vi "Process Intiation Response.vi"(5 "password":string, 7 "user name":string, 8 "error in (no error)":errorcluster, 9 "publicKeyB":u8[](array[numeric]), 10 "salt":u8[](array[numeric]), 11 "srp":T1) -> (0 "error out":errorcluster, 2 "clientHash":u8[](array[numeric]), 3 "srp":T1)   [LabVIEW 2016, in "SRP.lvlib"]
uses:
  <vilib>/addons/InsightCM/SRP/SRP.lvlib
  <vilib>/addons/InsightCM/SRP/controls/DVR_data.ctl
  <vilib>/addons/InsightCM/SRP/controls/data.ctl
  <vilib>/addons/InsightCM/SRP/libraries/win32Urelease/brsrp.dll
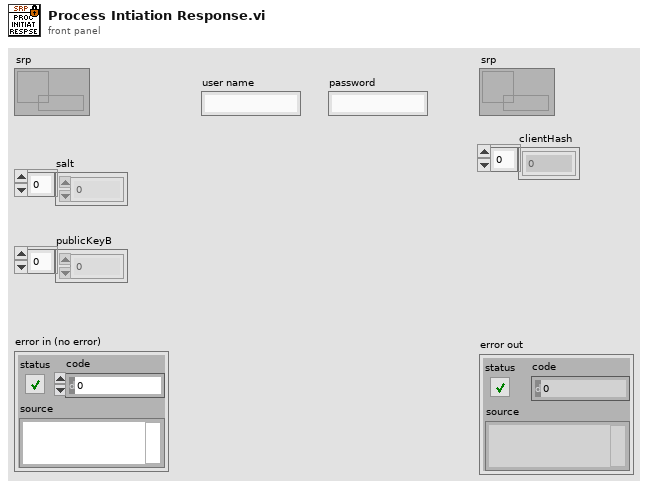
[diagram p1: front panel]
types:
  T1 = typedef "SRP.lvlib/DVR_data.ctl" = refnum<data-value>
  T2 = typedef "SRP.lvlib/data.ctl" = cluster{"SessionKey":u8[], "ClientHash":u8[], "PublicKeyA":u8[], "PrivateKeyA":u8[]}
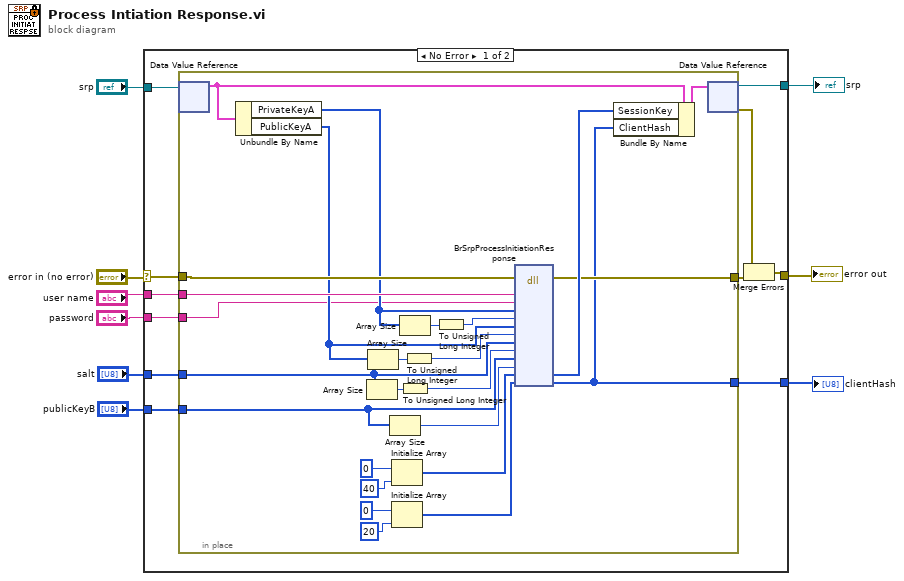
[diagram p0: block diagram]
diagram:
  n1 = case shown="No Error" "error in (no error)" {
    selector: "error in (no error)" -> [w16 w47]
    tunnel: [w19 w47] -> w9
    tunnel: "srp" -> [w20 w46]
    tunnel: "user name" -> [w15 _]
    tunnel: "password" -> [w14 _]
    tunnel: [w17 w46] -> w4
    tunnel: "salt" -> [w12 _]
    tunnel: "publicKeyB" -> [w11 _]
    tunnel: [w10 _] -> w1
    frame No Error {
      n2 = in-place {
        in-place-border: w16 -> [w35]
        in-place-border: w15 -> [w34]
        in-place-border: w14 -> [w21]
        in-place-border: [w32] -> w13
        in-place-border: w12 -> [w27]
        in-place-border: w11 -> [w31]
        in-place-border: [w30] -> w10
        n3 = in-place-dvr #1(w20) -> (w44:T2)  [unwired: 1 out]
        n4 = Unbundle By Name(w44) -> ("PrivateKeyA"=w23:u8[], "PublicKeyA"=w25:u8[])
        n5 = Array Size(array=w27) -> (size(s)=w43:i32)
        n6 = Array Size(array=w25) -> (size(s)=w28:i32)
        n7 = Array Size(array=w31) -> (size(s)=w42:i32)
        n8 = Initialize Array(u8 0, 40 ("dimension size")) -> (w37:u8[])
        n9 = Initialize Array(u8 0, 20 ("dimension size")) -> (w36:u8[])
        n10 = Array Size(array=w23) -> (size(s)=w24:i32)
        n11 = To Unsigned Long Integer(number=w43) -> (unsigned 32bit integer=w29:u32)
        n12 = To Unsigned Long Integer(number=w28) -> (unsigned 32bit integer=w26:u32)
        n13 = To Unsigned Long Integer(number=w24) -> (unsigned 32bit integer=w22:u32)
        n14 = dll-call lib="C:/Program Files (x86)/National Instruments/LabVIEW 2016/vi.lib/addons/InsightCM/SRP/libraries/win32Urelease/brsrp.*" fn="BrSrpProcessInitiationResponse"(error in=w35, "userName"=w34, "password"=w21, "privateKeyA"=w23, "privateKeyA_length"=w22, "publicKeyA"=w25, "publicKeyA_length"=w26, "salt"=w27, "salt_length"=w29, "publicKeyB"=w31, "publicKeyB_length"=w42, "sessionKey"=w37, "clientHash"=w36) -> (error out=w32:errorcluster, "sessionKey"=w33:u8[], "clientHash"=w30:u8[])  [unwired: 13 in, 1 out]
        n15 = Bundle By Name(cluster=w44, "SessionKey"=w33, "ClientHash"=w30) -> (w45:T2)
        n16 = in-place-dvr #1(w45) -> (w17:T1, w18:errorcluster)
      }
      n17 = Merge Errors(w18, w13) -> (w19:errorcluster)
    }
    frame Error {
    }
  }
  "error out" <- w9
  "srp" <- w4
  "clientHash" <- w1
